vi "Revision Query.vi"(8 "error in (no error)":errorcluster, 11 "VISA resource name":refnum<visa-resource-name>) -> (0 "error out":errorcluster, 1 "Instrument Firmware Revision":string, 2 "Instrument Driver Revision":string, 3 "VISA resource name out":refnum<visa-resource-name>)   [LabVIEW 2015, in "Micron Optics sm130.lvlib"]
doc: "Queries the current instrument firmware revision and instrument driver revision.\n\nRefer to the Readme file for detailed driver information including modification history."
uses:
  Micron Optics sm130.lvlib
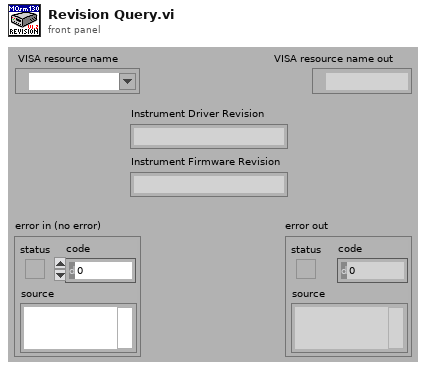
[diagram p1: front panel]
types:
  T1 = enum32{"invalid app kind", "Development System", "Run Time System", "Student Edition", "Embedded LabVIEW", "Evaluation", "Custom"}
  T2 = cluster{"Major":u16, "Minor":u16, "Fix":u16, "Build":u16}
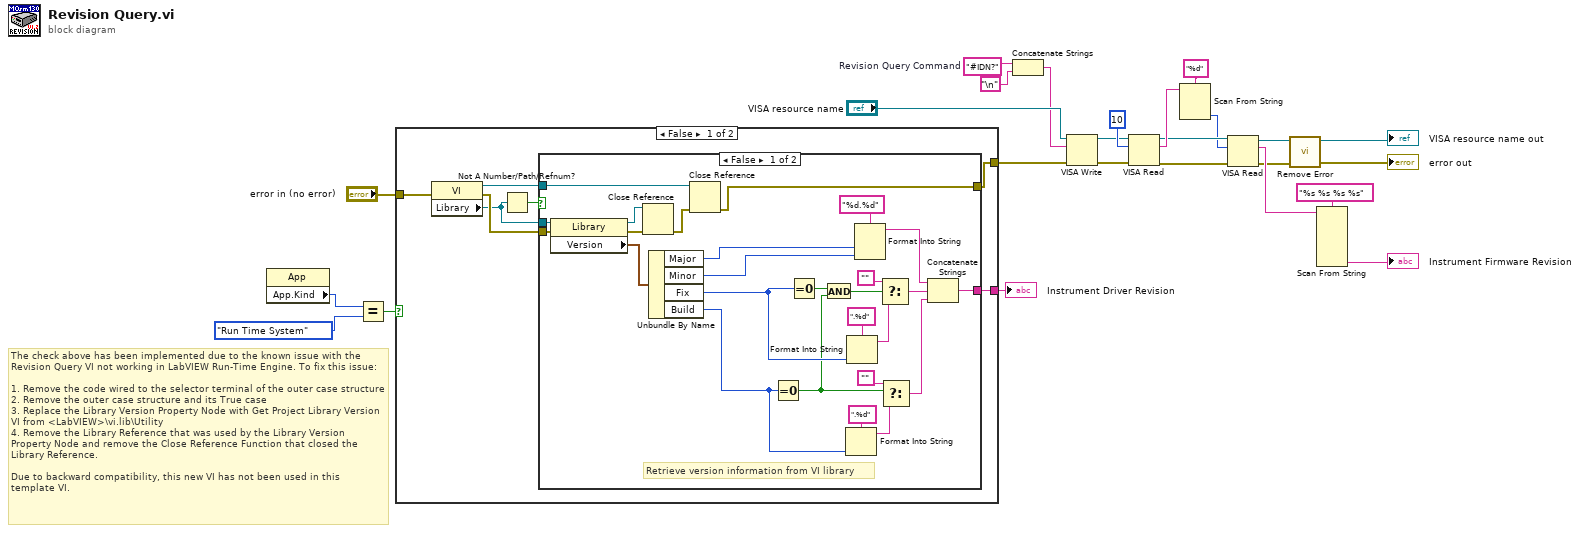
[diagram p0: block diagram]
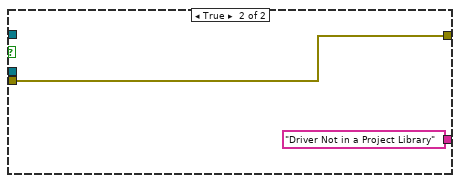
[diagram p2: hidden frame]
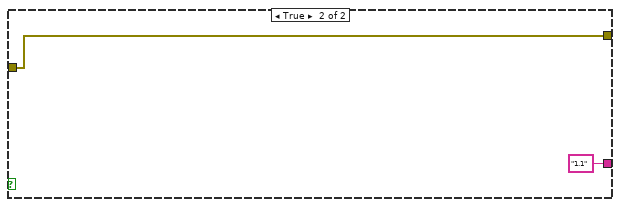
[diagram p3: hidden frame]
diagram:
  w8 = "#IDN?"  # Revision Query Command
  # "The check above has been implemented due to the known issue with the Revision Query VI not working in LabVIEW Run-Time Engine. To fix this issue:\n\n1. Remove the code wired to the selector terminal of the outer case structure\n2. Remove the outer case structure and its True case\n3. Replace the Library Version Property Node with Get Project Library Version VI from <LabVIEW>\\vi.lib\\Utility\n4. Remove the Library Reference that was used by the Library Version Property Node and remove the Close Reference Function that closed the Library Reference.\n\nDue to backward compatibility, this new VI has not been used in this template VI."
  n1 = property class="App"() -> ("App.Kind"=w16:T1)  [unwired: 2 in, 2 out]
  n2 = Equal?(x=w16, y=T1."Run Time System" ("Application:Kind")) -> (x = y?=w17:bool)
  n3 = case shown="False" w17 {
    tunnel: [w28 "1.1"] -> w20
    tunnel: "error in (no error)" -> [w27 w61]
    tunnel: [w26 w61] -> w18
    frame False {
      n4 = property class="VI"(error in=w27) -> (reference out=w32:refnum<vi>, error out=w31:errorcluster, "Library"=w30:refnum<vi>)  [unwired: 1 in]
      n5 = Not A Number/Path/Refnum?(number/path/refnum=w30) -> (NaN/Path/Refnum?=w29:bool)
      n6 = case shown="False" w29 {
        tunnel: w32 -> [w55 _]
        tunnel: w31 -> [w40 w60]
        tunnel: [w35 w60] -> w26
        tunnel: [w34 "Driver Not in a Project Library"] -> w28
        tunnel: w30 -> [w33 _]
        frame False {
          # "Retrieve version information from VI library"
          n7 = property class="Library"(reference=w33, error in=w40) -> (reference out=w57:refnum<vi>, error out=w58:errorcluster, "Version"=w54:T2)
          n8 = Close Reference(reference=w57, error in (no error)=w58) -> (error out=w56:errorcluster)
          n9 = Unbundle By Name(w54) -> ("Major"=w43:u16, "Minor"=w42:u16, "Fix"=w39:u16, "Build"=w41:u16)
          n10 = Close Reference(reference=w55, error in (no error)=w56) -> (error out=w35:errorcluster)
          n11 = Equal To 0?(x=w41) -> (x = 0?=w37:bool)
          n12 = Equal To 0?(x=w39) -> (x = 0?=w38:bool)
          n13 = And(x=w38, y=w37) -> (x .and. y?=w36:bool)
          n14 = Format Into String(format string=".%d", w41) -> (resulting string=w47:string)  [unwired: 2 in, 1 out]
          n15 = Format Into String(format string=".%d", w39) -> (resulting string=w51:string)  [unwired: 2 in, 1 out]
          n16 = Format Into String(format string="%d.%d", w43, w42) -> (resulting string=w49:string)  [unwired: 2 in, 1 out]
          n17 = Select(t="", s=w36, f=w51) -> (s? t:f=w48:string)
          n18 = Select(t="", s=w37, f=w47) -> (s? t:f=w44:string)
          n19 = Concatenate Strings(w49, w48, w44) -> (w34:string)
        }
        frame True {
        }
      }
    }
    frame True {
    }
  }
  "Instrument Driver Revision" <- w20
  n20 = Concatenate Strings(w8, "\n") -> (w6:string)
  n21 = VISA Write(VISA resource name="VISA resource name", write buffer=w6, error in (no error)=w18) -> (VISA resource name out=w22:refnum<visa-resource-name>, error out=w21:errorcluster)  [unwired: 1 out]
  n22 = VISA Read(VISA resource name=w22, byte count=u32 10 ("Bytes to Read"), error in (no error)=w21) -> (VISA resource name out=w12:refnum<visa-resource-name>, read buffer=w13:string, error out=w11:errorcluster)  [unwired: 1 out]
  n23 = Scan From String(format string="%d", input string=w13) -> (output 1=w10:i32)  [unwired: 3 in, 3 out]
  n24 = VISA Read(VISA resource name=w12, byte count=w10, error in (no error)=w11) -> (VISA resource name out=w4:refnum<visa-resource-name>, read buffer=w9:string, error out=w3:errorcluster)  [unwired: 1 out]
  n25 = call "Remove Error.vi"("error in (no error)"=w3, "VISA resource name"=w4) -> ("error out"=→"error out":errorcluster, "VISA resource name out"=→"VISA resource name out":refnum<visa-resource-name>)  [unwired: 8 in]
  n26 = Scan From String(format string="%s %s %s %s", input string=w9) -> (output 4=→"Instrument Firmware Revision":string)  [unwired: 9 in, 3 out]
